vi "SimpleStateMachineTemplate.vi"() -> ()   [LabVIEW 2020]
uses:
  State.ctl
panel:
  in  "Exit":bool
  in  "Stop":bool
  in  "Start":bool
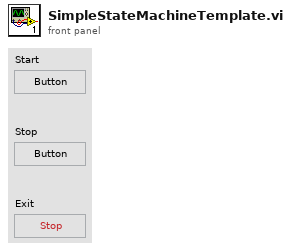
[diagram p1: front panel]
types:
  T1 = typedef "State.ctl" = enum16{"Exit", "Idle", "Stop", "Start", "Init"}
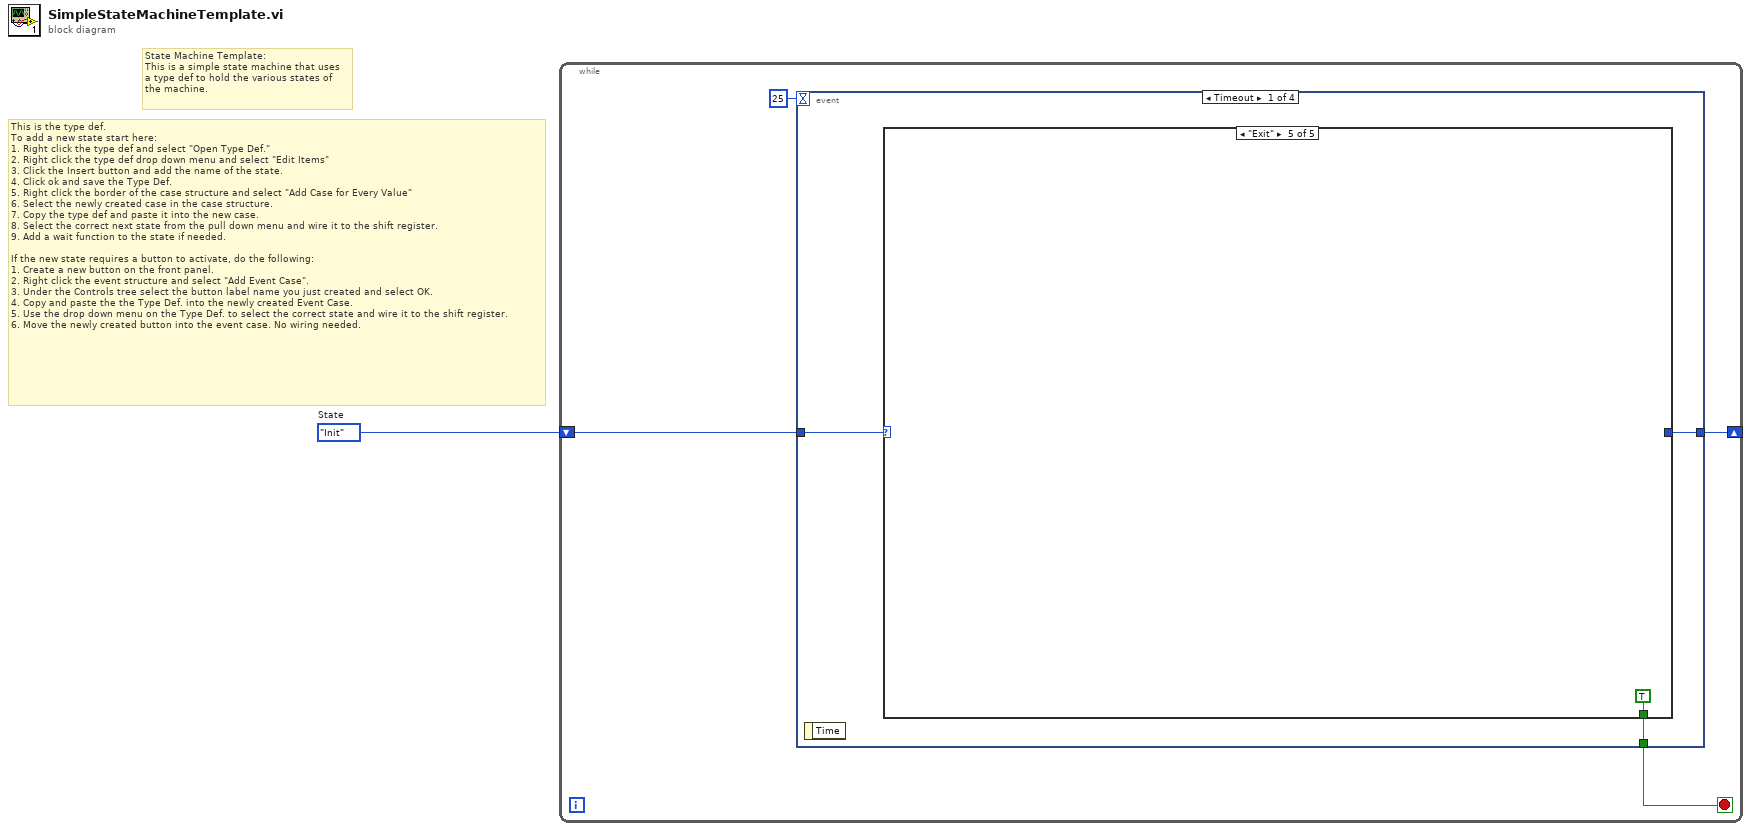
[diagram p0: block diagram]
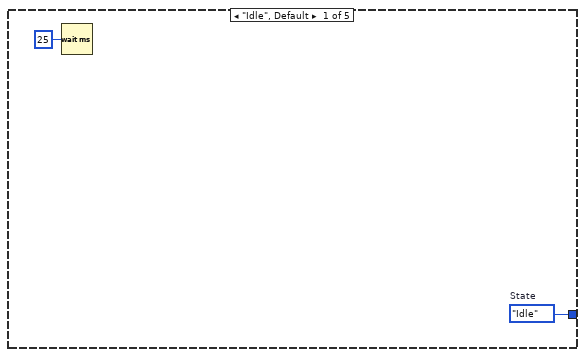
[diagram p2: hidden frame]
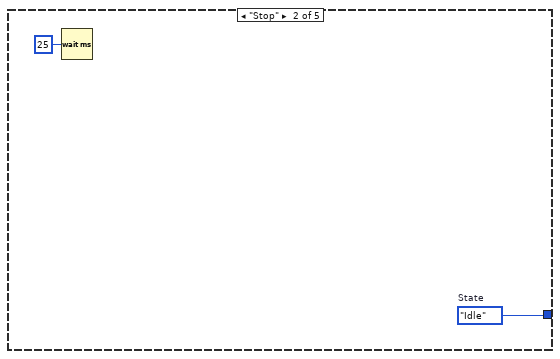
[diagram p3: hidden frame]
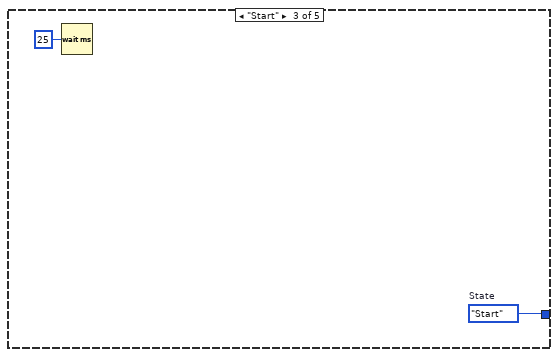
[diagram p4: hidden frame]
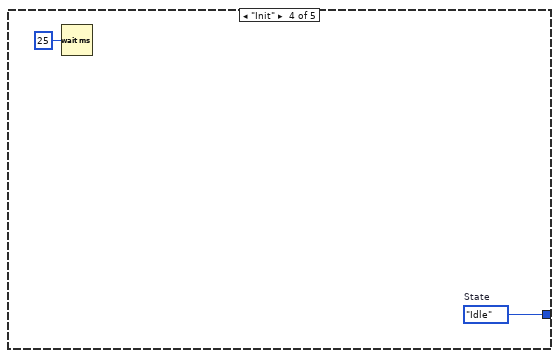
[diagram p5: hidden frame]
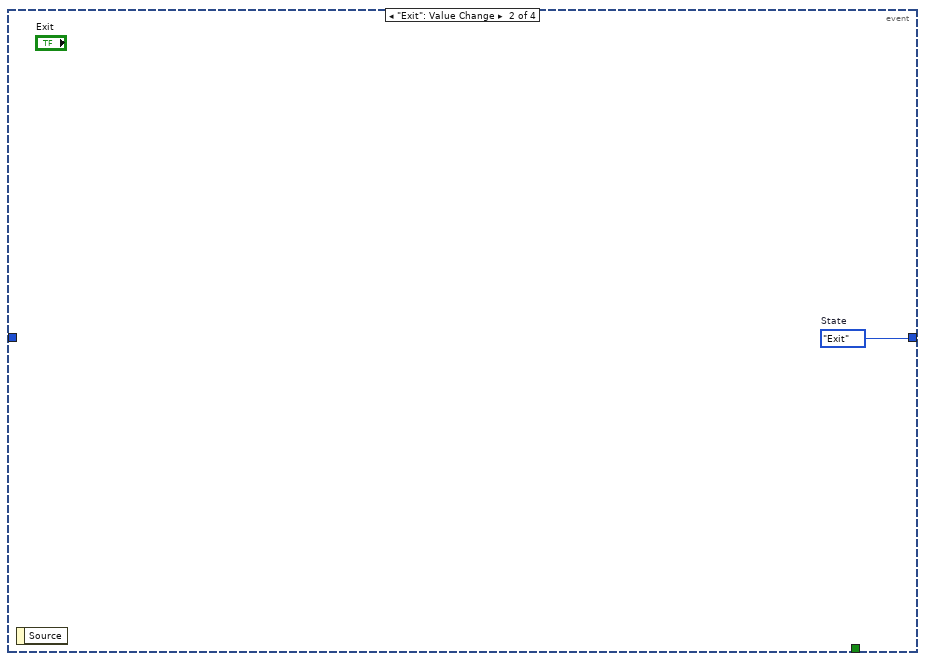
[diagram p6: hidden frame]
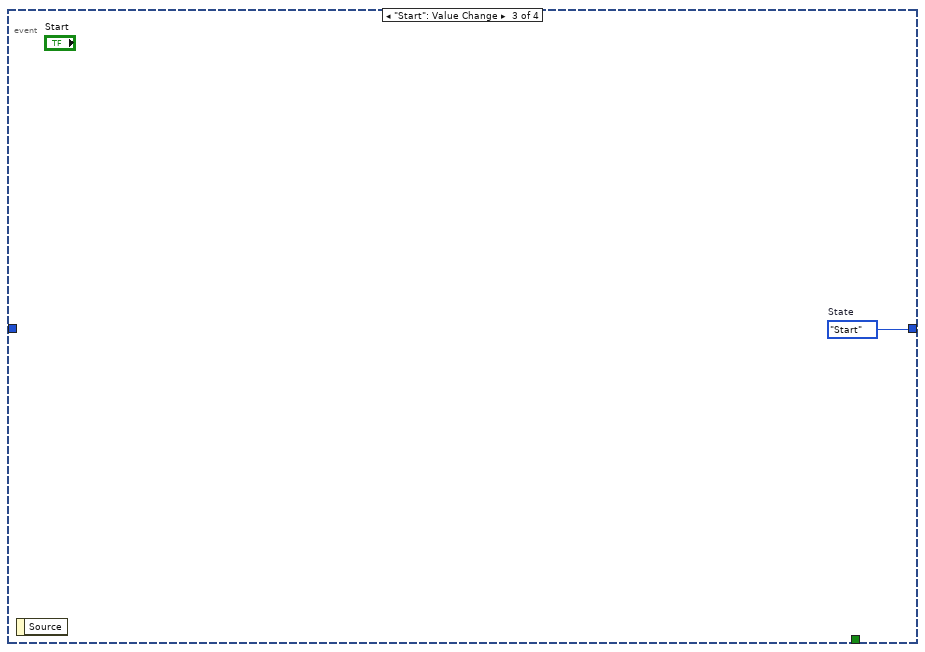
[diagram p7: hidden frame]
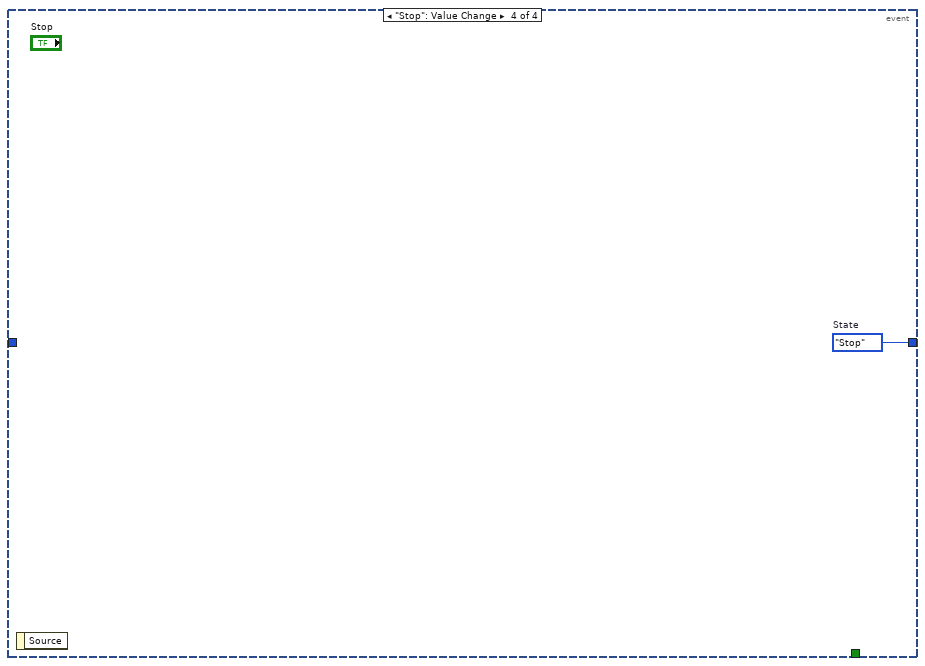
[diagram p8: hidden frame]
diagram:
  w1 = State."Init"  # State
  # "This is the type def.\nTo add a new state start here:\n1. Right click the type def and select \"Open Type Def.\"\n2. Right click the type def drop down menu and select \"Edit Items\"\n3. Click the Insert button and add the name of the state.\n4. Click ok and save the Type Def.\n5. Right click the border of the case structure and select \"Add Case for Every Value\"\n6. Select the newly created case in the case structure.\n7. Copy the type def and paste it into the new case.\n8. Select the correct next state from the pull down menu and wire it to the shift register.\n9. Add a wait function to the state if needed.\n\nIf the new state requires a button to activate, do the following:\n1. Create a new button on the front panel.\n2. Right click the event structure and select \"Add Event Case\".\n3. Under the Controls tree select the button label name you just created and select OK.\n4. Copy and paste the the Type Def. into the newly created Event Case.\n5. Use the drop down menu on the Type Def. to select the correct state and wire it to the shift register.\n6. Move the newly created button into the event case. No wiring needed."
  # "State Machine Template:\nThis is a simple state machine that uses\na type def to hold the various states of\nthe machine."
  n1 = while {
    shift-right: [w3] -> _
    shift-left: w1 -> [w4]
    stop <- w2 stop-if-true
    n2 = event shown="[0] Timeout" {
      selector: _ -> [_ _ _ _]
      dyn-events: _ -> [_ _ _ _]
      timeout: 25 -> [_ _ _ _]
      tunnel: w4 -> [w8 _ _ _]
      tunnel: [w7 w18 w19 w20] -> w3
      tunnel: [w6 _ _ _] -> w2
      event Timeout {
        n3 = event-data() -> ()  [unwired: 1 in, 1 out]
        n4 = case shown="\"Exit\"" w8 {
          tunnel: [w10 w12 w14 w16 _] -> w7
          tunnel: [_ _ _ _ TRUE] -> w6
          frame "Idle", Default {
            w10 = State."Idle"  # State
            n5 = Wait (ms)(milliseconds to wait=u32 25) -> ()  [unwired: 1 out]
          }
          frame "Stop" {
            w12 = State."Idle"  # State
            n6 = Wait (ms)(milliseconds to wait=u32 25) -> ()  [unwired: 1 out]
          }
          frame "Start" {
            w14 = State."Start"  # State
            n7 = Wait (ms)(milliseconds to wait=u32 25) -> ()  [unwired: 1 out]
          }
          frame "Init" {
            w16 = State."Idle"  # State
            n8 = Wait (ms)(milliseconds to wait=u32 25) -> ()  [unwired: 1 out]
          }
          frame "Exit" {
          }
        }
      }
      event "Exit": Value Change {
        w18 = State."Exit"  # State
        n9 = event-data() -> ()  [unwired: 1 in, 1 out]
      }
      event "Start": Value Change {
        w19 = State."Start"  # State
        n10 = event-data() -> ()  [unwired: 1 in, 1 out]
      }
      event "Stop": Value Change {
        w20 = State."Stop"  # State
        n11 = event-data() -> ()  [unwired: 1 in, 1 out]
      }
    }
  }
